vi "AuMT8852B EDR BER Floor Sensitivity Configuration.vi"(5 "Settings":T1={"Low frequency selection"=enum."Use low frequency", "Medium frequency selection"=enum."Use medium frequency", "High frequency selection"=enum."Use high frequency", "Low TX frequency"=2480.0, "Low RX frequency"=2402.0, "Medium TX frequency"=2402.0, "Medium RX frequency"=2441.0, "High TX frequency"=2402.0, "High RX frequency"=2480.0, "Threshold bit count"=0.1, "2DHx test packet"=enum."OFF", "3DHx test packet"=enum."OFF", "Hop selection"=enum."Test with hopping off and on", "Test TX power"=-70.0, "Packet count"=enum."TX", "Total test bit count"=0.1, "Threshold error limit (E-6)"=7, "Total test error limit (E-5)"=1} {"Total test bit count" format="%.2f"; "Test TX power" format="%.1f"; "Threshold bit count" format="%.2f"}, 7 "Set/Get (Set)":enum16{"Set", "Get"}(ring), 8 "error in (no error)":errorcluster, 10 "Script (3)":i32=3, 11 "VISA session":refnum<visa-resource-name>) -> (0 "error out":errorcluster, 2 "error code":i32, 3 "VISA session out":refnum<visa-resource-name>, 4 "Settings out":T1={"Low frequency selection"=enum."Use low frequency", "Medium frequency selection"=enum."Use medium frequency", "High frequency selection"=enum."Use high frequency", "Low TX frequency"=2480.0, "Low RX frequency"=2402.0, "Medium TX frequency"=2402.0, "Medium RX frequency"=2441.0, "High TX frequency"=2402.0, "High RX frequency"=2480.0, "Threshold bit count"=0.1, "2DHx test packet"=enum."OFF", "3DHx test packet"=enum."OFF", "Hop selection"=enum."Test with hopping off and on", "Test TX power"=-70.0, "Packet count"=enum."TX", "Total test bit count"=0.1, "Threshold error limit (E-6)"=7, "Total test error limit (E-5)"=1} {"Total test bit count" format="%.2f"; "Test TX power" format="%.1f"; "Threshold bit count" format="%.2f"})   [LabVIEW 2017]
doc: "Anritsu MT8852B Bluetooth Tester\n\nConfigures the instrument for the EDR BER Floor Sensitivity test.\n\nINPUTS\nSet/Get - whether the values are being sent to or retrieved from the instrument.\nScript - which of the stored scripts (1-10) will be queried or configured. Scripts 1 and 2 are read-only.\nSettings - parameters of the test to be written.\n\nOUTPUTS\nSettings out - current parameters of the test."
uses:
  <instrlib>/aumt8852B/General/Utilities/MT8850 Test Parameters.ctl
  <instrlib>/aumt8852B/General/Utilities/MT8850 Frequency Units.ctl
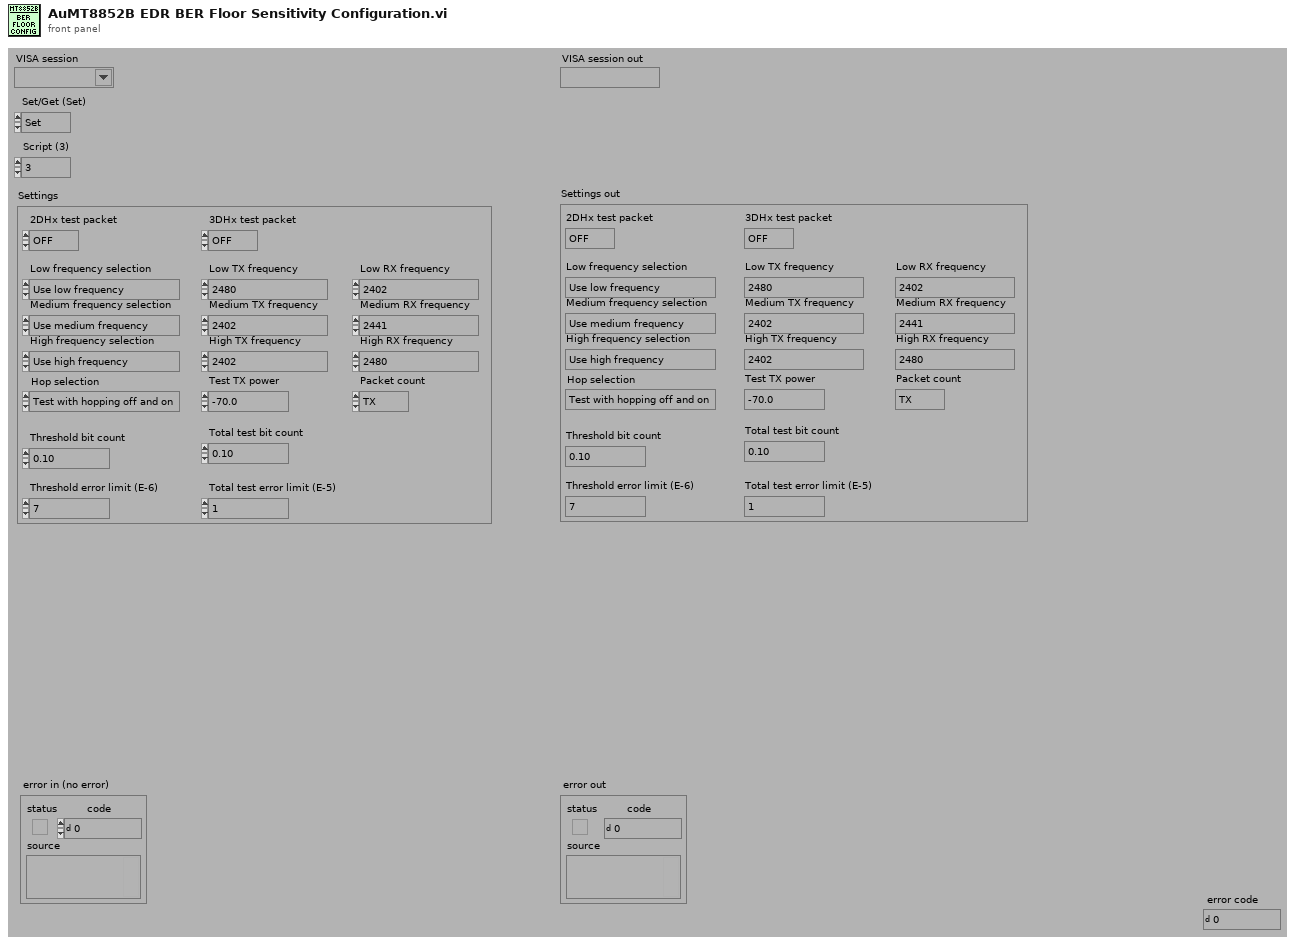
[diagram p1: front panel]
types:
  T1 = cluster{"Low frequency selection":enum16{"Don't use low frequency", "Use low frequency"}, "Medium frequency selection":enum16{"Don't use medium frequency", "Use medium frequency"}, "High frequency selection":enum16{"Don't use high frequency", "Use high frequency"}, "Low TX frequency":dbl, "Low RX frequency":dbl, "Medium TX frequency":dbl, "Medium RX frequency":dbl, "High TX frequency":dbl, "High RX frequency":dbl, "Threshold bit count":dbl, "2DHx test packet":enum16{"OFF", "Longest", "2-DH1", "2-DH3", "2-DH5"}, "3DHx test packet":enum16{"OFF", "Longest", "3-DH1", "3-DH3", "3-DH5"}, "Hop selection":enum16{"Test with hopping on", "Test with hopping off", "Test with hopping off and on"}, "Test TX power":dbl, "Packet count":enum16{"TX", "RX"}, "Total test bit count":dbl, "Threshold error limit (E-6)":i16, "Total test error limit (E-5)":i16}
  T2 = typedef "MT8850 Test Parameters.ctl" = enum16{"Use low frequency", "Use medium frequency", "Use high frequency", "Low TX frequency", "Low RX frquency", "Medium TX frequency", "Medium RX frequency", "High TX frequency", "High RX frequency", "Number of packets", "Average high limit", "Average low limit", "Peak power limit", "Max power step limit", "Min power step limit", "f1 average minimum", "f1 average maximum", "f2 maximum", "f1/f2 average maximum", "Hop selection", "Use DH1 packets", "Use DH3 packets", "Use DH5 packets", "1 slot packet drift limit", "3 slot packet drift limit", "5 slot packet drift limit", "Drift rate limit", "TX power level", "Frequency offset", "Symbol timing", "Modulation index", "BER limit", "FER limit", "Use averaging high limit", "Use averaging low limit", "Use peak power limit", "Packet type", "Test control", "Use max power step limit", "Use min power step limit", "Number of cycles", "Use f1 average maximum", "Use f1 average minimum", "Use f2 maximum", "Use f1/f2 average maximum", "Hop mode", "Maximum negative limit", "Maximum positive limit", "Use maximum negative limit", "Use maximum positive limit", "Use 1 slot packet drift limit", "Use 3 slot packet drift limit", "Use 5 slot packet drift limit", "Use drift rate limit", "Use BER limit", "Use FER limit", "Use dirty parameter table", "Use null packet drift limit", "Null packet drift limit", "Minimum power", "Power delay", "Packet count", "Payload toggle", "Output power level", "2DHX packet type", "3DHX packet type", "Number of blocks", "TX and RX low frequency", "TX and RX medium frequency", "TX and RX high frequency", "TX frequency", "RX frequency", "Threshold bit count", "Total test bit count", "Number of bits", "PDPSK to PGFSK lower limit", "PDPSK to PGFSK upper limit", "Initial frequency error upper limit", "Initial frequency error lower limit", "Frequency error upper limit", "Frequency error lower limit", "Block frequency error upper limit", "Block frequency error lower limit", "2Mbs RMS DEVM limit", "3Mbs RMS DEVM limit", "2Mbs Peak DEVM limit", "3Mbs Peak DEVM limit", "2Mbs 99% packets DEVM limit", "3Mbs 99% packets DEVM limit", "Percentage of no error packets limit", "Threshold error limit", "Total test error limit"}
  T3 = enum16{"Output power", "Power control", "Modulation characteristics", "Initial carrier", "Carrier drift", "Single slot sensitivity", "Multiple slot sensitivity", "Maximum input power", "EDR Relative transmit power", "EDR Carrier frequency and stability", "EDR Differential phase encoding", "EDR Sensitivity", "EDR BER floor sensitivity", "EDR Maximum input power"}
  T4 = typedef "MT8850 Frequency Units.ctl" = enum16{"Channel", "Hz", "kHz", "MHz", "GHz"}
  T5 = enum16{"Simulate", "Range check", "Cache", "Query instrument status"}
  T6 = enum16{"Test with hopping on", "Test with hopping off", "Test with hopping off and on"}
  T7 = enum16{"OFF", "Longest", "3-DH1", "3-DH3", "3-DH5"}
  T8 = enum16{"OFF", "Longest", "2-DH1", "2-DH3", "2-DH5"}
  T9 = enum16{"Don't use high frequency", "Use high frequency"}
  T10 = enum16{"Don't use medium frequency", "Use medium frequency"}
  T11 = enum16{"Don't use low frequency", "Use low frequency"}
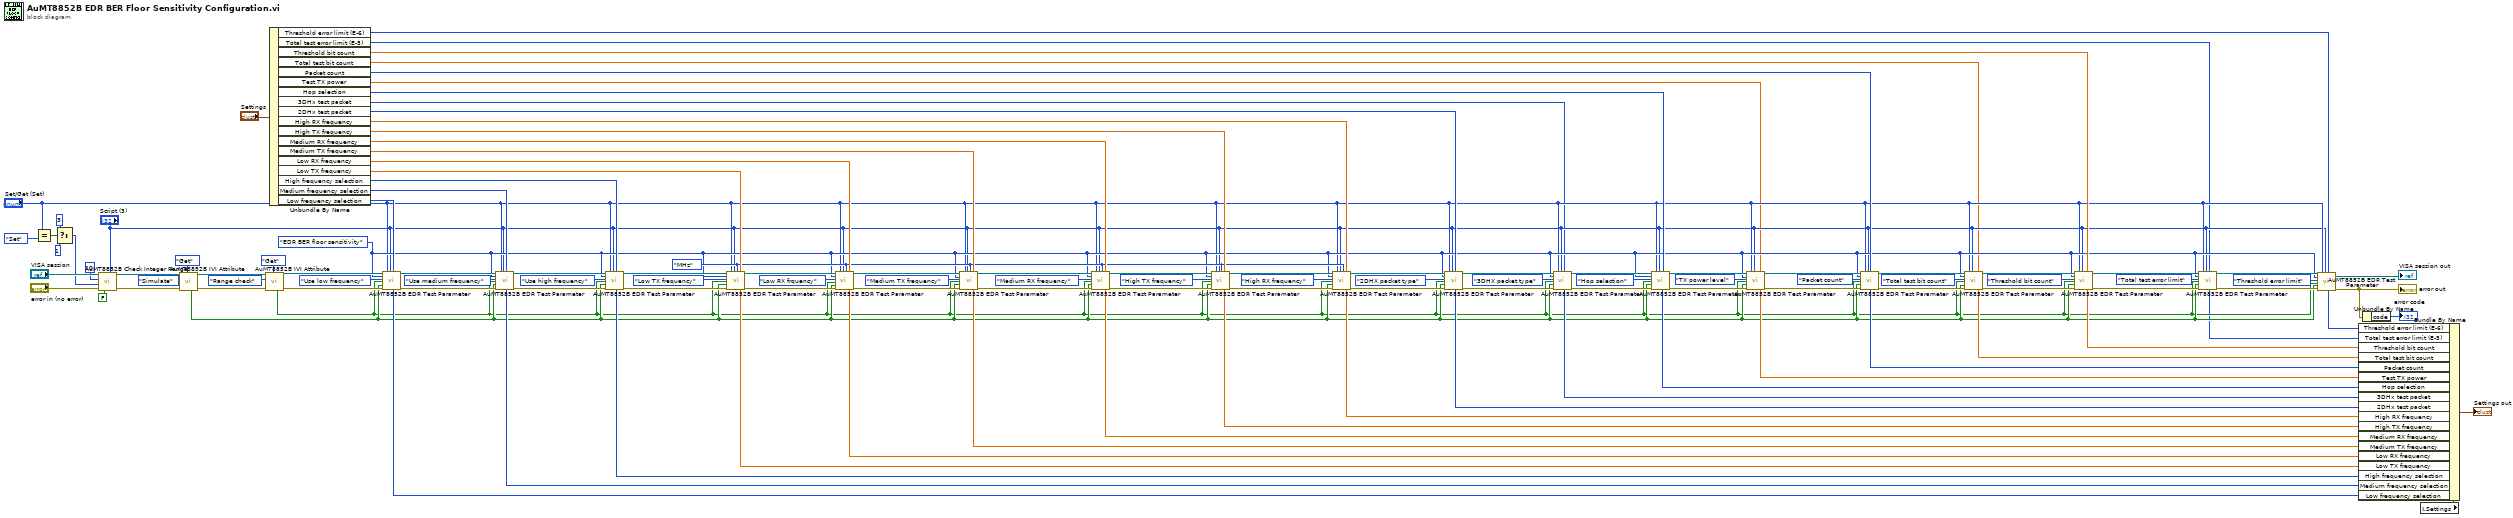
[diagram p0: block diagram]
diagram:
  w11 = T3."EDR BER floor sensitivity" ("Test (Output power)")
  w47 = MT8850_Frequency_Units."MHz" ("Frequency units (MHz)")
  n1 = Equal?(x="Set/Get (Set)", y=enum16{"Set", "Get"}."Set") -> (x = y?=w116:bool)
  n2 = Select(t=3, s=w116, f=1) -> (s? t:f=w112:i32)
  n3 = call <instrlib>:"AuMT8852B Check Integer Range.vi"("Value (0)"="Script (3)", "Check IVI flag first? (T)"=FALSE, "error in (no error)"="error in (no error)", "Lower limit (-1)"=w112, "Upper limit (1)"=10, "VISA session"="VISA session") -> ("error out"=w110:errorcluster, "VISA session out"=w111:refnum<visa-resource-name>)  [unwired: 4 in]
  n4 = call <instrlib>:"AuMT8852B IVI Attribute.vi"("Set/Get (Set)"=enum16{"Set", "Get"}."Get", "error in (no error)"=w110, "Flag (Simulate)"=T5."Simulate", "VISA session"=w111) -> ("error out"=w84:errorcluster, "VISA session out"=w85:refnum<visa-resource-name>, "Value out"=w17:bool)  [unwired: 5 in]
  n5 = call <instrlib>:"AuMT8852B IVI Attribute.vi"("Set/Get (Set)"=enum16{"Set", "Get"}."Get", "error in (no error)"=w84, "Flag (Simulate)"=T5."Range check", "VISA session"=w85) -> ("error out"=w82:errorcluster, "VISA session out"=w83:refnum<visa-resource-name>, "Value out"=w16:bool)  [unwired: 5 in]
  n6 = Unbundle By Name("Settings") -> ("Threshold error limit (E-6)"=w3:i16, "Total test error limit (E-5)"=w4:i16, "Threshold bit count"=w25:dbl, "Total test bit count"=w7:dbl, "Packet count"=w32:enum16{"TX", "RX"}, "Test TX power"=w6:dbl, "Hop selection"=w38:T6, "3DHx test packet"=w5:T7, "2DHx test packet"=w60:T8, "High RX frequency"=w72:dbl, "High TX frequency"=w73:dbl, "Medium RX frequency"=w61:dbl, "Medium TX frequency"=w74:dbl, "Low RX frequency"=w75:dbl, "Low TX frequency"=w76:dbl, "High frequency selection"=w77:T9, "Medium frequency selection"=w78:T10, "Low frequency selection"=w79:T11)
  n7 = call <instrlib>:"AuMT8852B EDR Test Parameter.vi"("VISA session"=w83, "Test (Output power)"=w11, "Parameter (Use low frequency)"=MT8850_Test_Parameters."Use low frequency", "Range check? (F)"=w16, "Simulate? (F)"=w17, "error in (no error)"=w82, "Set/Get (Set)"="Set/Get (Set)", "Script (3)"="Script (3)", "Integer value (0)"=w79) -> ("Integer value out"=w64:i32, "VISA session out"=w53:refnum<visa-resource-name>, "error out"=w52:errorcluster)  [unwired: 7 in, 1 out]
  n8 = call <instrlib>:"AuMT8852B EDR Test Parameter.vi"("VISA session"=w53, "Test (Output power)"=w11, "Parameter (Use low frequency)"=MT8850_Test_Parameters."Use medium frequency", "Range check? (F)"=w16, "Simulate? (F)"=w17, "error in (no error)"=w52, "Set/Get (Set)"="Set/Get (Set)", "Script (3)"="Script (3)", "Integer value (0)"=w78) -> ("Integer value out"=w65:i32, "VISA session out"=w51:refnum<visa-resource-name>, "error out"=w50:errorcluster)  [unwired: 7 in, 1 out]
  n9 = call <instrlib>:"AuMT8852B EDR Test Parameter.vi"("VISA session"=w51, "Test (Output power)"=w11, "Parameter (Use low frequency)"=MT8850_Test_Parameters."Use high frequency", "Range check? (F)"=w16, "Simulate? (F)"=w17, "error in (no error)"=w50, "Set/Get (Set)"="Set/Get (Set)", "Script (3)"="Script (3)", "Integer value (0)"=w77) -> ("Integer value out"=w66:i32, "VISA session out"=w106:refnum<visa-resource-name>, "error out"=w105:errorcluster)  [unwired: 7 in, 1 out]
  n10 = call <instrlib>:"AuMT8852B EDR Test Parameter.vi"("VISA session"=w106, "Test (Output power)"=w11, "Parameter (Use low frequency)"=MT8850_Test_Parameters."Low TX frequency", "Range check? (F)"=w16, "Simulate? (F)"=w17, "error in (no error)"=w105, "Set/Get (Set)"="Set/Get (Set)", "Script (3)"="Script (3)", "Integer value (0)"=w47, "Float value (0)"=w76) -> ("Float value out"=w67:dbl, "VISA session out"=w104:refnum<visa-resource-name>, "error out"=w103:errorcluster)  [unwired: 6 in, 1 out]
  n11 = call <instrlib>:"AuMT8852B EDR Test Parameter.vi"("VISA session"=w104, "Test (Output power)"=w11, "Parameter (Use low frequency)"=MT8850_Test_Parameters."Low RX frquency", "Range check? (F)"=w16, "Simulate? (F)"=w17, "error in (no error)"=w103, "Set/Get (Set)"="Set/Get (Set)", "Script (3)"="Script (3)", "Integer value (0)"=w47, "Float value (0)"=w75) -> ("Float value out"=w68:dbl, "VISA session out"=w102:refnum<visa-resource-name>, "error out"=w101:errorcluster)  [unwired: 6 in, 1 out]
  n12 = call <instrlib>:"AuMT8852B EDR Test Parameter.vi"("VISA session"=w102, "Test (Output power)"=w11, "Parameter (Use low frequency)"=MT8850_Test_Parameters."Medium TX frequency", "Range check? (F)"=w16, "Simulate? (F)"=w17, "error in (no error)"=w101, "Set/Get (Set)"="Set/Get (Set)", "Script (3)"="Script (3)", "Integer value (0)"=w47, "Float value (0)"=w74) -> ("Float value out"=w69:dbl, "VISA session out"=w100:refnum<visa-resource-name>, "error out"=w99:errorcluster)  [unwired: 6 in, 1 out]
  n13 = call <instrlib>:"AuMT8852B EDR Test Parameter.vi"("VISA session"=w100, "Test (Output power)"=w11, "Parameter (Use low frequency)"=MT8850_Test_Parameters."Medium RX frequency", "Range check? (F)"=w16, "Simulate? (F)"=w17, "error in (no error)"=w99, "Set/Get (Set)"="Set/Get (Set)", "Script (3)"="Script (3)", "Integer value (0)"=w47, "Float value (0)"=w61) -> ("Float value out"=w63:dbl, "VISA session out"=w98:refnum<visa-resource-name>, "error out"=w97:errorcluster)  [unwired: 6 in, 1 out]
  n14 = call <instrlib>:"AuMT8852B EDR Test Parameter.vi"("VISA session"=w98, "Test (Output power)"=w11, "Parameter (Use low frequency)"=MT8850_Test_Parameters."High TX frequency", "Range check? (F)"=w16, "Simulate? (F)"=w17, "error in (no error)"=w97, "Set/Get (Set)"="Set/Get (Set)", "Script (3)"="Script (3)", "Integer value (0)"=w47, "Float value (0)"=w73) -> ("Float value out"=w70:dbl, "VISA session out"=w96:refnum<visa-resource-name>, "error out"=w95:errorcluster)  [unwired: 6 in, 1 out]
  n15 = call <instrlib>:"AuMT8852B EDR Test Parameter.vi"("VISA session"=w96, "Test (Output power)"=w11, "Parameter (Use low frequency)"=MT8850_Test_Parameters."High RX frequency", "Range check? (F)"=w16, "Simulate? (F)"=w17, "error in (no error)"=w95, "Set/Get (Set)"="Set/Get (Set)", "Script (3)"="Script (3)", "Integer value (0)"=w47, "Float value (0)"=w72) -> ("Float value out"=w71:dbl, "VISA session out"=w94:refnum<visa-resource-name>, "error out"=w93:errorcluster)  [unwired: 6 in, 1 out]
  n16 = call <instrlib>:"AuMT8852B EDR Test Parameter.vi"("VISA session"=w94, "Test (Output power)"=w11, "Parameter (Use low frequency)"=MT8850_Test_Parameters."2DHX packet type", "Range check? (F)"=w16, "Simulate? (F)"=w17, "error in (no error)"=w93, "Set/Get (Set)"="Set/Get (Set)", "Script (3)"="Script (3)", "Integer value (0)"=w60) -> ("Integer value out"=w62:i32, "VISA session out"=w56:refnum<visa-resource-name>, "error out"=w55:errorcluster)  [unwired: 7 in, 1 out]
  n17 = call <instrlib>:"AuMT8852B EDR Test Parameter.vi"("VISA session"=w56, "Test (Output power)"=w11, "Parameter (Use low frequency)"=MT8850_Test_Parameters."3DHX packet type", "Range check? (F)"=w16, "Simulate? (F)"=w17, "error in (no error)"=w55, "Set/Get (Set)"="Set/Get (Set)", "Script (3)"="Script (3)", "Integer value (0)"=w5) -> ("Integer value out"=w31:i32, "VISA session out"=w41:refnum<visa-resource-name>, "error out"=w42:errorcluster)  [unwired: 7 in, 1 out]
  n18 = call <instrlib>:"AuMT8852B EDR Test Parameter.vi"("VISA session"=w41, "Test (Output power)"=w11, "Parameter (Use low frequency)"=MT8850_Test_Parameters."Hop selection", "Range check? (F)"=w16, "Simulate? (F)"=w17, "error in (no error)"=w42, "Set/Get (Set)"="Set/Get (Set)", "Script (3)"="Script (3)", "Integer value (0)"=w38) -> ("Integer value out"=w30:i32, "VISA session out"=w40:refnum<visa-resource-name>, "error out"=w43:errorcluster)  [unwired: 7 in, 1 out]
  n19 = call <instrlib>:"AuMT8852B EDR Test Parameter.vi"("VISA session"=w40, "Test (Output power)"=w11, "Parameter (Use low frequency)"=MT8850_Test_Parameters."TX power level", "Range check? (F)"=w16, "Simulate? (F)"=w17, "error in (no error)"=w43, "Set/Get (Set)"="Set/Get (Set)", "Script (3)"="Script (3)", "Float value (0)"=w6) -> ("Float value out"=w22:dbl, "VISA session out"=w35:refnum<visa-resource-name>, "error out"=w37:errorcluster)  [unwired: 7 in, 1 out]
  n20 = call <instrlib>:"AuMT8852B EDR Test Parameter.vi"("VISA session"=w35, "Test (Output power)"=w11, "Parameter (Use low frequency)"=MT8850_Test_Parameters."Packet count", "Range check? (F)"=w16, "Simulate? (F)"=w17, "error in (no error)"=w37, "Set/Get (Set)"="Set/Get (Set)", "Script (3)"="Script (3)", "Integer value (0)"=w32) -> ("Integer value out"=w29:i32, "VISA session out"=w34:refnum<visa-resource-name>, "error out"=w36:errorcluster)  [unwired: 7 in, 1 out]
  n21 = call <instrlib>:"AuMT8852B EDR Test Parameter.vi"("VISA session"=w34, "Test (Output power)"=w11, "Parameter (Use low frequency)"=MT8850_Test_Parameters."Total test bit count", "Range check? (F)"=w16, "Simulate? (F)"=w17, "error in (no error)"=w36, "Set/Get (Set)"="Set/Get (Set)", "Script (3)"="Script (3)", "Float value (0)"=w7) -> ("Float value out"=w24:dbl, "VISA session out"=w46:refnum<visa-resource-name>, "error out"=w45:errorcluster)  [unwired: 7 in, 1 out]
  n22 = call <instrlib>:"AuMT8852B EDR Test Parameter.vi"("VISA session"=w46, "Test (Output power)"=w11, "Parameter (Use low frequency)"=MT8850_Test_Parameters."Threshold bit count", "Range check? (F)"=w16, "Simulate? (F)"=w17, "error in (no error)"=w45, "Set/Get (Set)"="Set/Get (Set)", "Script (3)"="Script (3)", "Float value (0)"=w25) -> ("Float value out"=w23:dbl, "VISA session out"=w27:refnum<visa-resource-name>, "error out"=w28:errorcluster)  [unwired: 7 in, 1 out]
  n23 = call <instrlib>:"AuMT8852B EDR Test Parameter.vi"("VISA session"=w27, "Test (Output power)"=w11, "Parameter (Use low frequency)"=MT8850_Test_Parameters."Total test error limit", "Range check? (F)"=w16, "Simulate? (F)"=w17, "error in (no error)"=w28, "Set/Get (Set)"="Set/Get (Set)", "Script (3)"="Script (3)", "Integer value (0)"=w4) -> ("Integer value out"=w1:i32, "VISA session out"=w18:refnum<visa-resource-name>, "error out"=w19:errorcluster)  [unwired: 7 in, 1 out]
  n24 = call <instrlib>:"AuMT8852B EDR Test Parameter.vi"("VISA session"=w18, "Test (Output power)"=w11, "Parameter (Use low frequency)"=MT8850_Test_Parameters."Threshold error limit", "Range check? (F)"=w16, "Simulate? (F)"=w17, "error in (no error)"=w19, "Set/Get (Set)"="Set/Get (Set)", "Script (3)"="Script (3)", "Integer value (0)"=w3) -> ("Integer value out"=w2:i32, "VISA session out"=→"VISA session out":refnum<visa-resource-name>, "error out"=w12:errorcluster)  [unwired: 7 in, 1 out]
  "error out" <- w12
  n25 = Unbundle By Name(w12) -> ("code"=→"error code":i32)
  n26 = local read "Settings"() -> (w21:T1)
  n27 = Bundle By Name(cluster=w21, "Threshold error limit (E-6)"=w2, "Total test error limit (E-5)"=w1, "Threshold bit count"=w23, "Total test bit count"=w24, "Packet count"=w29, "Test TX power"=w22, "Hop selection"=w30, "3DHx test packet"=w31, "2DHx test packet"=w62, "High RX frequency"=w71, "High TX frequency"=w70, "Medium RX frequency"=w63, "Medium TX frequency"=w69, "Low RX frequency"=w68, "Low TX frequency"=w67, "High frequency selection"=w66, "Medium frequency selection"=w65, "Low frequency selection"=w64) -> (→"Settings out":T1)
